vi "Split text with format.vi"(2 "error in (no error)":errorcluster, 3 "Str Refnum":refnum<vi>) -> (0 "error out":errorcluster, 1 "String and format [ ]":T1(array[cluster]))   [LabVIEW 2019]
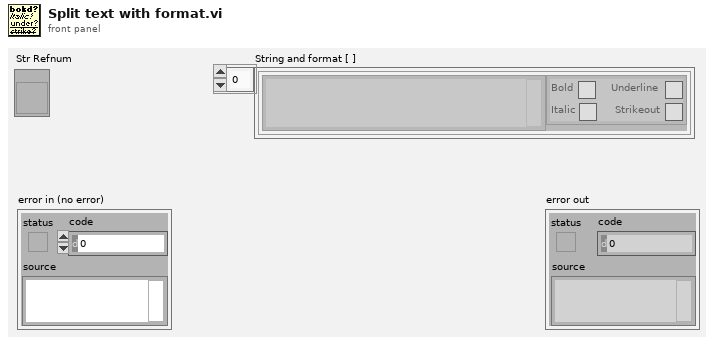
[diagram p1: front panel]
types:
  T1 = cluster{"string":string, "Style":cluster{"Bold":bool, "Italic":bool, "Underline":bool, "Strikeout":bool}}[]
  T2 = cluster{"Bold":bool, "Italic":bool, "Underline":bool, "Strikeout":bool}
  T3 = cluster{string, "Style":cluster{"Bold":bool, "Italic":bool, "Underline":bool, "Strikeout":bool}}[]
  T4 = cluster{"Text.FontBold":bool, "Text.FontItalic":bool, "Text.FontUnder":bool, "Text.FontStrike":bool}
  T5 = cluster{"Value":string, "Style":cluster{"Text.FontBold":bool, "Text.FontItalic":bool, "Text.FontUnder":bool, "Text.FontStrike":bool}}
  T6 = cluster{"Value":string, "Style":cluster{"Text.FontBold":bool, "Text.FontItalic":bool, "Text.FontUnder":bool, "Text.FontStrike":bool}}[]
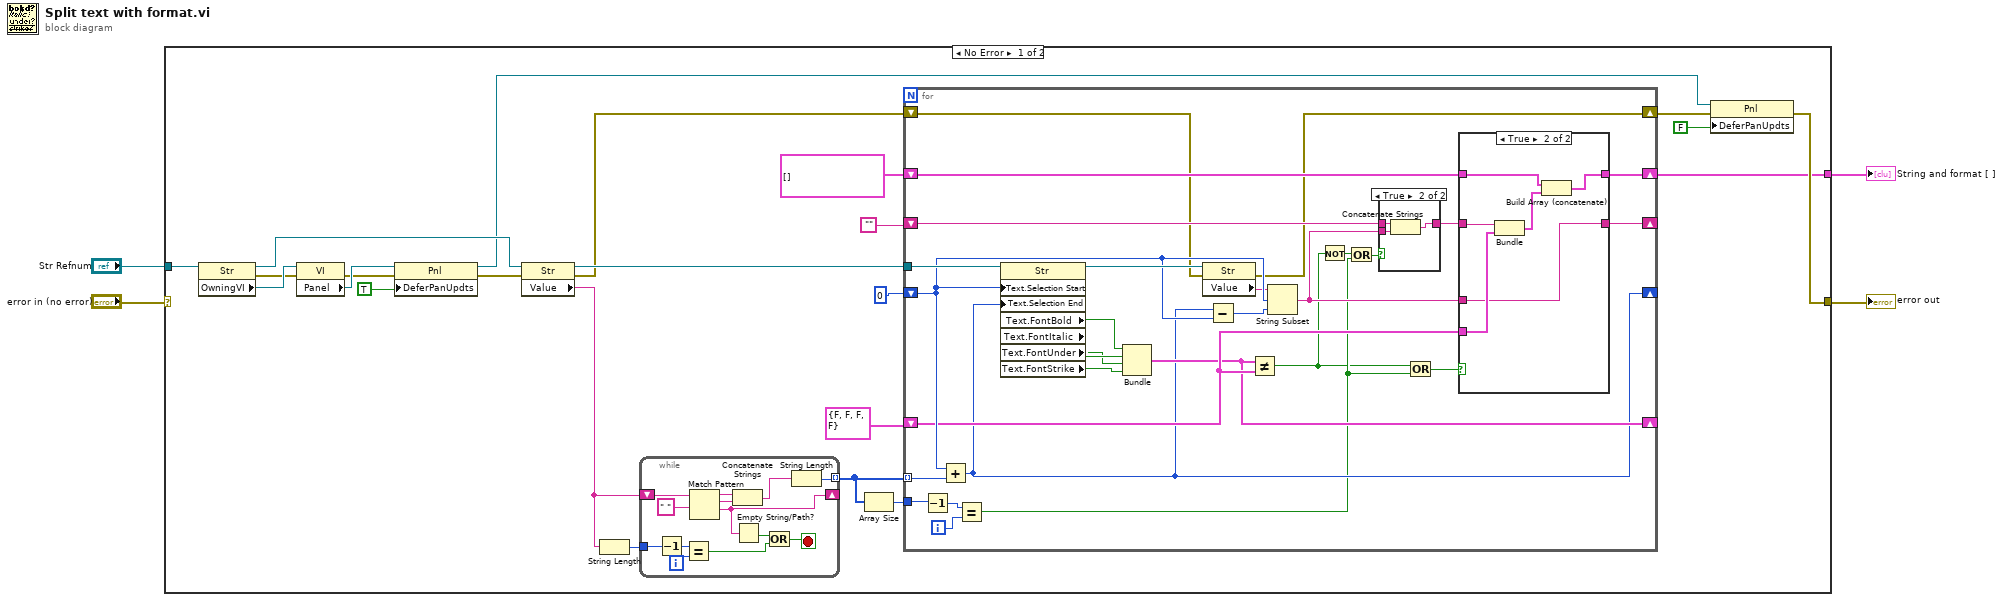
[diagram p0: block diagram]
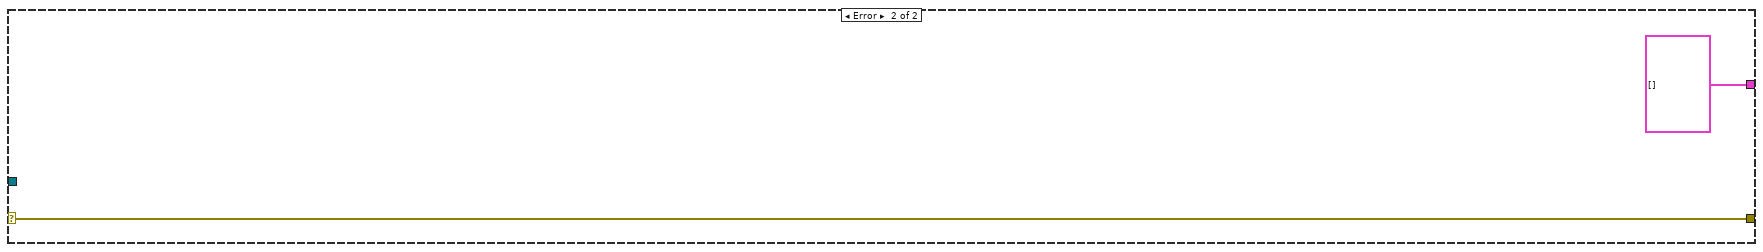
[diagram p4: hidden frame]
diagram:
  n1 = case shown="No Error" "error in (no error)" {
    selector: "error in (no error)" -> [_ w83]
    tunnel: [w25 T3 []] -> w4
    tunnel: "Str Refnum" -> [w15 _]
    tunnel: [w27 w83] -> w1
    frame No Error {
      n2 = property class="Str"(reference=w15) -> (reference out=w17:refnum<vi>, error out=w18:errorcluster, "OwningVI"=w22:refnum<vi>)  [unwired: 1 in]
      n3 = property class="VI"(reference=w22, error in=w18) -> (error out=w20:errorcluster, "Panel"=w21:refnum<vi>)  [unwired: 1 out]
      n4 = property class="Pnl"(reference=w21, error in=w20, "DeferPanUpdts"=TRUE ("Defer Panel Updates")) -> (reference out=w11:refnum<vi>, error out=w16:errorcluster)
      n5 = property class="Str"(reference=w17, error in=w16) -> (reference out=w24:refnum<vi>, error out=w13:errorcluster, "Value"=w8:string)
      n6 = String Length(string=w8) -> (length=w7:i32)
      n7 = while {
        shift-right: [w36] -> _
        shift-left: w8 -> [w40]
        tunnel: w7 -> [w32]
        tunnel: [w29] -> w6 mode=indexing
        i -> [w33]
        stop <- w35 stop-if-true
        n8 = Decrement(x=w32) -> (x-1=w31:i32)
        n9 = Equal?(x=w31, y=w33) -> (x = y?=w30:bool)
        n10 = Match Pattern(string=w40, regular expression=" ") -> (before substring=w38:string, match substring=w37:string, after substring=w36:string)  [unwired: 2 out]
        n11 = Concatenate Strings(w38, w37) -> (w28:string)
        n12 = Empty String/Path?(string/path=w36) -> (empty?=w34:bool)
        n13 = Or(x=w34, y=w30) -> (x .or. y?=w35:bool)
        n14 = String Length(string=w28) -> (length=w29:i32)
      }
      n15 = Array Size(array=w6) -> (size(s)=w5:i32)
      n16 = for {
        tunnel: w24 -> [w69]
        shift-right: [w67] -> w25
        shift-left: T3 [] -> [w68]
        shift-right: [w54] -> _
        shift-left: 0 -> [w65]
        tunnel: w6 -> [w64] mode=indexing
        shift-right: [w55] -> _
        shift-left: T2 {"Bold"=FALSE, "Italic"=FALSE, "Underline"=FALSE, "Strikeout"=FALSE} ("Style") -> [w57]
        shift-right: [w56] -> _
        shift-left: "" -> [w48]
        tunnel: w5 -> [w53]
        shift-right: [w41] -> w12
        shift-left: w13 -> [w42]
        i -> [w51]
        n17 = Decrement(x=w53) -> (x-1=w52:i32)
        n18 = Add(x=w65, y=w64) -> (x+y=w54:i32)
        n19 = Equal?(x=w52, y=w51) -> (x = y?=w46:bool)
        n20 = property class="Str"(reference=w69, "Text.Selection Start"=w65, "Text.Selection End"=w54) -> (reference out=w66:refnum<vi>, "Text.FontBold"=w63:bool, "Text.FontItalic"=w62:bool, "Text.FontUnder"=w61:bool, "Text.FontStrike"=w60:bool)  [unwired: 1 in, 1 out]
        n21 = Bundle("Text.FontBold"=w63, "Text.FontItalic"=w62, "Text.FontUnder"=w61, "Text.FontStrike"=w60) -> (w55:T4)  [unwired: 1 out]
        n22 = property class="Str"(reference=w66, error in=w42) -> (error out=w41:errorcluster, "Value"=w59:string)  [unwired: 1 out]
        n23 = Subtract(x=w54, y=w65) -> (x-y=w58:i32)
        n24 = Not Equal?(x=w55, y=w57) -> (x != y?=w43:bool)
        n25 = String Subset(string=w59, offset (0)=w65, length (rest)=w58) -> (substring=w47:string)
        n26 = Not(x=w43) -> (.not. x?=w44:bool)
        n27 = Or(x=w44, y=w46) -> (x .or. y?=w45:bool)
        n28 = case shown="True" w45 {
          tunnel: [w70 w73] -> w49
          tunnel: w48 -> [w70 w72]
          tunnel: w47 -> [_ w71]
          frame False {
          }
          frame True {
            n29 = Concatenate Strings(w72, w71) -> (w73:string)
          }
        }
        n30 = Or(x=w43, y=w46) -> (x .or. y?=w50:bool)
        n31 = case shown="True" w50 {
          tunnel: w68 -> [w75 w81]
          tunnel: [w75 w80] -> w67
          tunnel: w57 -> [_ w79]
          tunnel: [w74 w77] -> w56
          tunnel: w47 -> [_ w77]
          tunnel: w49 -> [w74 w76]
          frame False {
          }
          frame True {
            n32 = Bundle("Value"=w76, "Style"=w79) -> (w78:T5)  [unwired: 1 out]
            n33 = Build Array (concatenate)(w81, w78) -> (w80:T6)
          }
        }
      }
      n34 = property class="Pnl"(reference=w11, error in=w12, "DeferPanUpdts"=FALSE ("Defer Panel Updates")) -> (error out=w27:errorcluster)  [unwired: 1 out]
    }
    frame Error {
    }
  }
  "String and format [ ]" <- w4
  "error out" <- w1
